vi "json Delete - array path.vi"(8 "error in (no error)":errorcluster, 10 "path":string, 11 "JSON Document in":refnum<class "JSON Document.lvclass">) -> (0 "error out":errorcluster, 3 "JSON Document out":refnum<class "JSON Document.lvclass">)   [LabVIEW 2015, in "JSON Document.lvclass"]
uses:
  JSON Document.lvclass
  JSON Document.lvclass/JSON Document.ctl
  rapidjson wrapper/rapidjson wrapper.lvlib
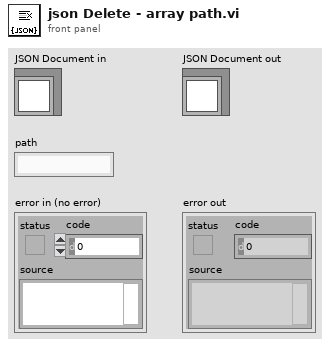
[diagram p1: front panel]
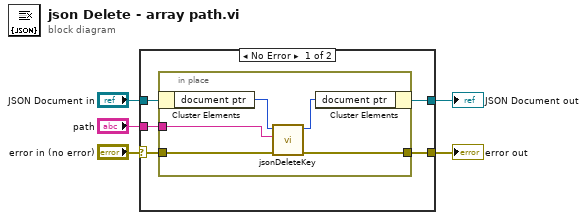
[diagram p0: block diagram]
diagram:
  n1 = case shown="No Error" "error in (no error)" {
    selector: "error in (no error)" -> [w7 w17]
    tunnel: [w6 w17] -> w4
    tunnel: [w9 w16] -> w2
    tunnel: "JSON Document in" -> [w10 w16]
    tunnel: "path" -> [w8 _]
    frame No Error {
      n2 = in-place {
        in-place-border: w8 -> [w13]
        in-place-border: w7 -> [w12]
        in-place-border: [w11] -> w6
        n3 = in-place-cluster #1(w10) -> ("document ptr"=w15:i64)
        n4 = call "jsonDeleteKey.vi"("error in (no error)"=w12, "path"=w13, "d in"=w15) -> ("error out"=w11:errorcluster, "d out"=w14:i64)  [unwired: 7 in]
        n5 = in-place-cluster #1("document ptr"=w14) -> (w9:refnum<class "JSON Document.lvclass">)
      }
    }
    frame Error {
    }
  }
  "error out" <- w4
  "JSON Document out" <- w2
